vi "PWM_output_SW-timed_with_digital_line (vers 8.2).vi"() -> ()   [LabVIEW 2016]
doc: "INSTRUCTIONS:\nThis Vi generates a software-timed PWM using one digital line as output:\n1. Select the digital line you want to use as output of your PWM.\n2. Introduce the Cycle time of the PWM signal.\n3. Select the accuracy (number of steps in a cycle).\n4. Select the duty cycle (in %) and the idle state (resting state of the output terminal)\n5. Every time a cycle is finished new values are loaded.\n6. Press the STOP switch to finish generation"
uses:
  <vilib>/Utility/error.llb/DialogType.ctl
  <vilib>/DAQmx/write.llb/DAQmx Write (Digital 1D Bool 1Chan 1Samp).vi
  <vilib>/DAQmx/miscellaneous.llb/DAQmx Fill In Error Info.vi
  <vilib>/DAQmx/create/channels.llb/DAQmx Create Channel (DO-Digital Output).vi
panel:
  in  "Idle State":bool
  out "Output":i16(graph)
  in  "Duty cycle % (0-100)":dbl=50.0
  in  "Cycle time PWM (seconds)":i32=5
  in  "Steps in a cycle":i32=256
  in  "Lines":tag="Dev1/port0/line0:7" caption="Digital output line"
  in  "STOP":bool
  # "PWM Configuration"
  # "INSTRUCTIONS:\nThis Vi generates a software-timed PWM using one digital line as output:\n1. Select the digital line you want to use as output of your PWM.\n2. Introduce the Cycle time of the PWM signal.\n3. Select the accuracy (number of steps in a cycle).\n4. Select the duty cycle (in %) and the idle state (resting state of the output terminal)\n5. Every time a cycle is finished new values are loaded.\n6. Press the STOP switch to finish generation."
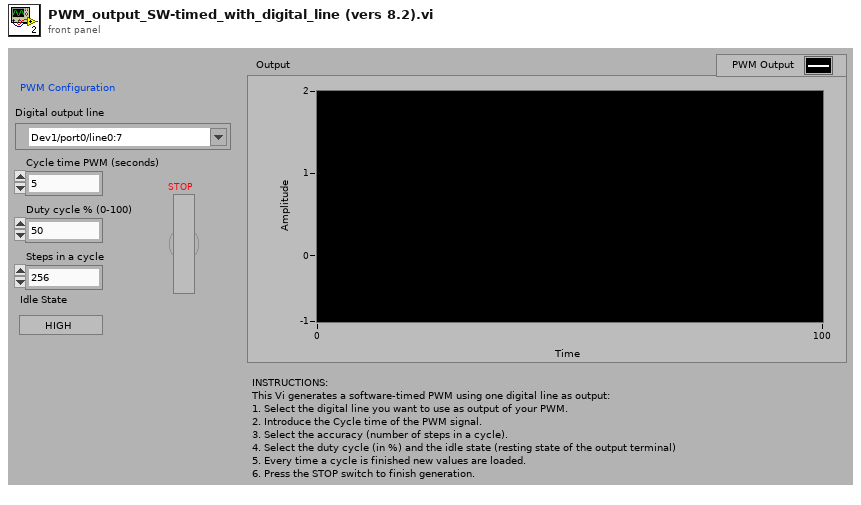
[diagram p1: front panel]
types:
  T1 = typedef "DialogType.ctl" = u16
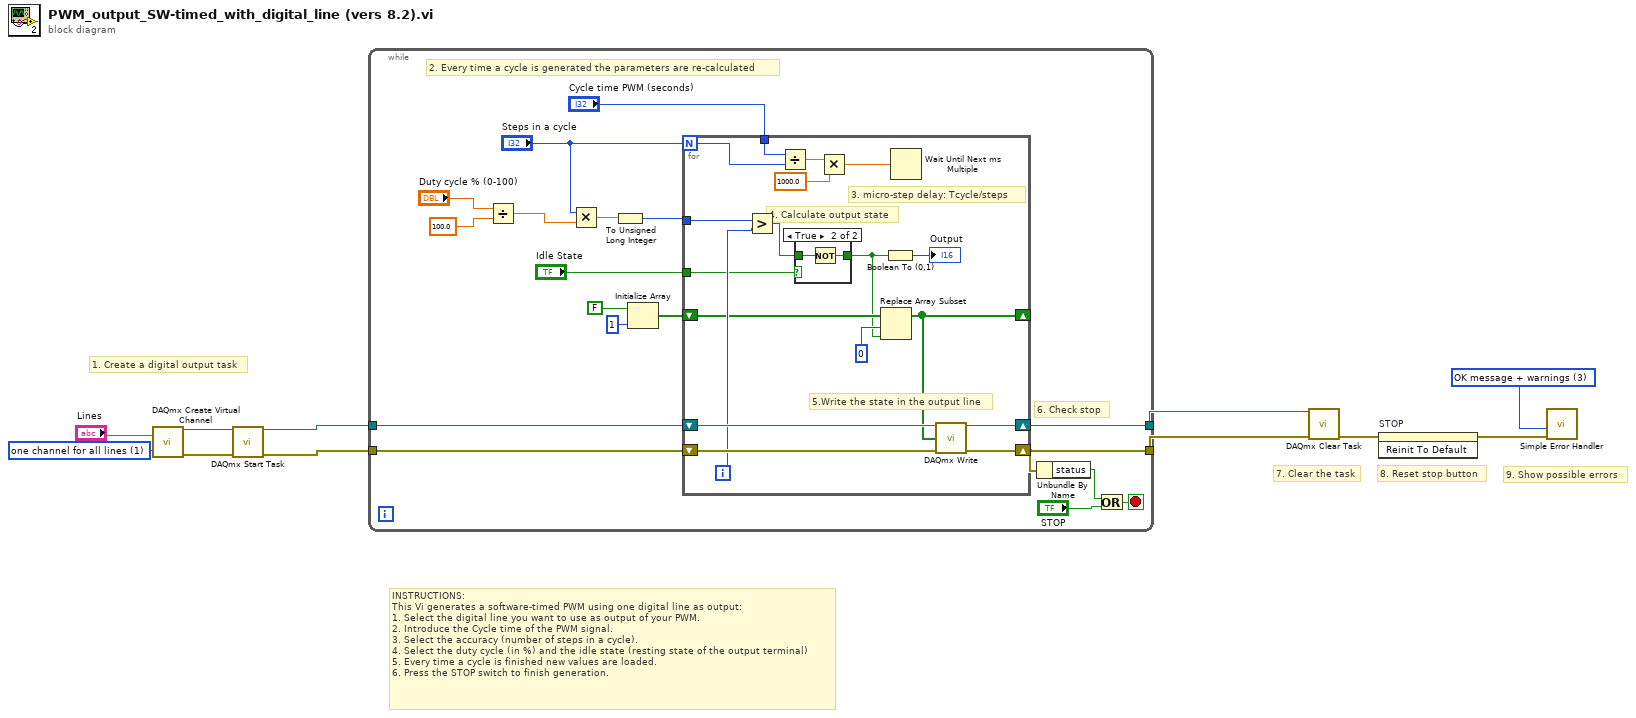
[diagram p0: block diagram]
diagram:
  w7 = 1 items=["one channel for each line", "one channel for all lines"] ("line grouping")
  w8 = T1 3 items=["no dialog", "OK message", "continue or stop message", "OK message + warnings", "continue/stop + warnings"] ("type of dialog (OK msg:1)")
  # "9. Show possible errors"
  # "8. Reset stop button"
  # "7. Clear the task"
  # "1. Create a digital output task"
  # "INSTRUCTIONS:\nThis Vi generates a software-timed PWM using one digital line as output:\n1. Select the digital line you want to use as output of your PWM.\n2. Introduce the Cycle time of the PWM signal.\n3. Select the accuracy (number of steps in a cycle).\n4. Select the duty cycle (in %) and the idle state (resting state of the output terminal)\n5. Every time a cycle is finished new values are loaded.\n6. Press the STOP switch to finish generation."
  n1 = call-poly <vilib>:"DAQmx Create Virtual Channel.vi"("lines"="Lines", "line grouping"=w7) -> ("task out"=w11:refnum<k21>, "error out"=w10:errorcluster)  [unwired: 12 in]
  n2 = call <vilib>:"DAQmx Start Task.vi"("task/channels in"=w11, "error in"=w10) -> ("task out"=w4:refnum<k21>, "error out"=w3:errorcluster)  [unwired: 12 in]
  n3 = while {
    tunnel: [w25] -> w6
    tunnel: [w16] -> w5
    tunnel: w4 -> [w24]
    tunnel: w3 -> [w23]
    stop <- w13 stop-if-true
    # "6. Check stop"
    # "2. Every time a cycle is generated the parameters are re-calculated"
    n4 = Divide(x="Duty cycle % (0-100)", y=100.0) -> (x/y=w26:dbl)
    n5 = Multiply(x="Steps in a cycle", y=w26) -> (x*y=w18:dbl)
    n6 = To Unsigned Long Integer(number=w18) -> (unsigned 32bit integer=w17:u32)
    n7 = Initialize Array(FALSE, 1 ("dimension size")) -> (w20:bool[])
    n8 = for {
      N: "Steps in a cycle" -> [w46]
      tunnel: "Cycle time PWM (seconds)" -> [w47]
      tunnel: w17 -> [w43]
      shift-right: [w42] -> w25
      shift-left: w24 -> [w39]
      shift-right: [w41] -> w16
      shift-left: w23 -> [w40]
      shift-right: [w33] -> _
      shift-left: w20 -> [w35]
      tunnel: "Idle State" -> [w32]
      i -> [w36]
      # "5.Write the state in the output line"
      # "4. Calculate output state"
      # "3. micro-step delay: Tcycle/steps"
      n9 = Greater?(x=w43, y=w36) -> (0:w31:bool)
      n10 = Divide(x=w47, y=w46) -> (x/y=w45:dbl)
      n11 = case shown="True" w32 {
        tunnel: [w48 w49] -> w30
        tunnel: w31 -> [w48 w50]
        frame False {
        }
        frame True {
          n12 = Not(x=w50) -> (.not. x?=w49:bool)
        }
      }
      n13 = Multiply(x=w45, y=1000.0) -> (x*y=w38:dbl)
      n14 = Replace Array Subset(array=w35, new element=w30, index=0) -> (w33:bool[])
      n15 = Boolean To (0,1)(Boolean=w30) -> (0, 1=→"Output":i16)
      n16 = Wait Until Next ms Multiple(millisecond multiple=w38) -> ()  [unwired: 1 out]
      n17 = call-poly <vilib>:"DAQmx Write.vi"("task/channels in"=w39, "data"=w33, "error in"=w40) -> ("task out"=w42:refnum<k21>, "error out"=w41:errorcluster)  [unwired: 10 in, 1 out]
    }
    n18 = Unbundle By Name(w16) -> ("status"=w15:bool)
    n19 = Or(x=w15, y="STOP") -> (x .or. y?=w13:bool)
  }
  n20 = call <vilib>:"DAQmx Clear Task.vi"("task in"=w6, "error in"=w5) -> ("error out"=w2:errorcluster)  [unwired: 13 in]
  n21 = invoke on="STOP" class="Bool (strict)" method="Reinit To Default"(error in=w2) -> (error out=w1:errorcluster)  [unwired: 2 in, 2 out]
  n22 = call <vilib>:"Simple Error Handler.vi"("type of dialog (OK msg:1)"=w8, "error in (no error)"=w1) -> ()  [unwired: 3 in, 5 out]
